vi "Initial Date Yields.vi"(8 "error in (no error)":errorcluster, 11 "Master in":refnum<class "Master.lvclass">) -> (0 "error out":errorcluster, 3 "Master out":refnum<class "Master.lvclass">)   [LabVIEW 2014, in "Master.lvclass"]
uses:
  Master/Master.lvclass
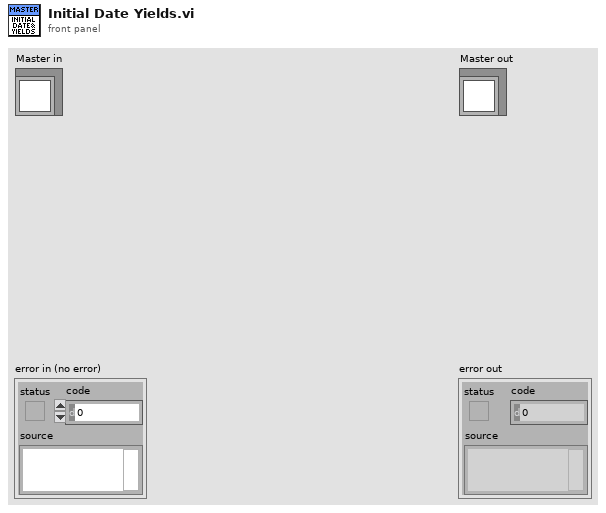
[diagram p1: front panel]
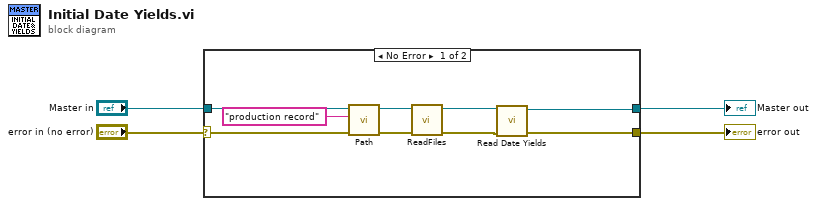
[diagram p0: block diagram]
diagram:
  n1 = case shown="No Error" "error in (no error)" {
    selector: "error in (no error)" -> [w7 w15]
    tunnel: [w6 w15] -> w3
    tunnel: [w8 w14] -> w1
    tunnel: "Master in" -> [w13 w14]
    frame No Error {
      n2 = call-dynamic "Path.vi"("error in (no error)"=w7, "pathname"="production record", "Master in"=w13) -> ("error out"=w11:errorcluster, "Master out"=w12:refnum<class "Master.lvclass">)  [unwired: 7 in]
      n3 = call-dynamic "ReadFiles.vi"("error in (no error)"=w11, "Master in"=w12) -> ("error out"=w9:errorcluster, "Master out"=w10:refnum<class "Master.lvclass">)  [unwired: 8 in]
      n4 = call-dynamic "Read Date Yields.vi"("error in (no error)"=w9, "Master in"=w10) -> ("error out"=w6:errorcluster, "Master out"=w8:refnum<class "Master.lvclass">)  [unwired: 8 in]
    }
    frame Error {
    }
  }
  "error out" <- w3
  "Master out" <- w1
